vi "YFM11.vi"() -> ()   [LabVIEW 2017]
uses:
  <vilib>/Analysis/6fits.llb/Curve Fitting Criteria.ctl
  <vilib>/DAQmx/write.llb/DAQmx Write (Analog DBL 1Chan 1Samp).vi
  <vilib>/DAQmx/read.llb/DAQmx Read (Analog Wfm 1Chan NSamp).vi
  <vilib>/DAQmx/create/channels.llb/DAQmx Create Channel (AO-Voltage-Basic).vi
  <vilib>/DAQmx/create/channels.llb/DAQmx Create Channel (AI-Voltage-Basic).vi
  <vilib>/DAQmx/configure/timing.llb/DAQmx Timing (Sample Clock).vi
  <vilib>/DAQmx/miscellaneous.llb/DAQmx Fill In Error Info.vi
  <vilib>/Analysis/6fits.llb/1D B-Spline Fit.vi
  <vilib>/Analysis/NI_AALPro.lvlib
panel:
  in  "averaging points":i32=100
  in  "sensitivity^-1":dbl=1000.0
  out "(log)Id(Vg)":cluster{dbl[], "Best BSpline Fit Y":dbl[]}(graph)
  out "intercept":dbl=nan
  out "theta avg.":dbl
  in  "stop":dbl=1.39
  in  "start":dbl=1.39
  out "theta":dbl[](array[numeric])
  in  "theta0":dbl
  out "Rct":dbl=nan
  out "YFM":dbl[](array[numeric])
  out "Vg":dbl[](array[numeric])
  in  "stop":dbl=1.4
  in  "start":dbl=1.1
  out "(Gm)^1/2":dbl=nan
  out "Vt":dbl=nan
  out "theta":cluster{dbl[], dbl[]}(graph)={[0.8, 0.81, 0.8200000000000001, 0.8300000000000001, 0.8400000000000001], [nan, nan, nan, nan, nan]}
  out "YFM":cluster{dbl[], "Best Linear Fit":dbl[]}(graph)
  out "gm":cluster{dbl[], dbl[]}(graph)={[0.8, 0.81, 0.8200000000000001, 0.8300000000000001, 0.8400000000000001], [-1.462188767798153e-07, 1.7166614532470683e-06, 3.266596794128415e-06, 2.5996923446655253e-06, -6.398235458925546e-08]}
  out "Id Array":dbl[](array[numeric])=[-1.173257827758789e-07, -1.1843729019165039e-07, -8.29925537109375e-08, -5.3105354309082036e-08, -3.099870681762695e-08]
  out "Vg Array":dbl[](array[numeric])=[0.8, 0.81, 0.8200000000000001, 0.8300000000000001, 0.8400000000000001]
  in  "Vd":dbl=0.1
  in  "Vd channels":tag="Dev3/ao1"
  in  "Id channels":tag="Dev9/ai0"
  out "# of step":dbl=60.999999999999986
  in  "Step":dbl=0.01
  in  "Stop (V)":dbl=1.4
  in  "Start (V)":dbl=0.8
  in  "Vg channels":tag="Dev3/ao0"
  # "<theta range>"
  # "<linear region>"
  # "Vg"
  # "Fitting"
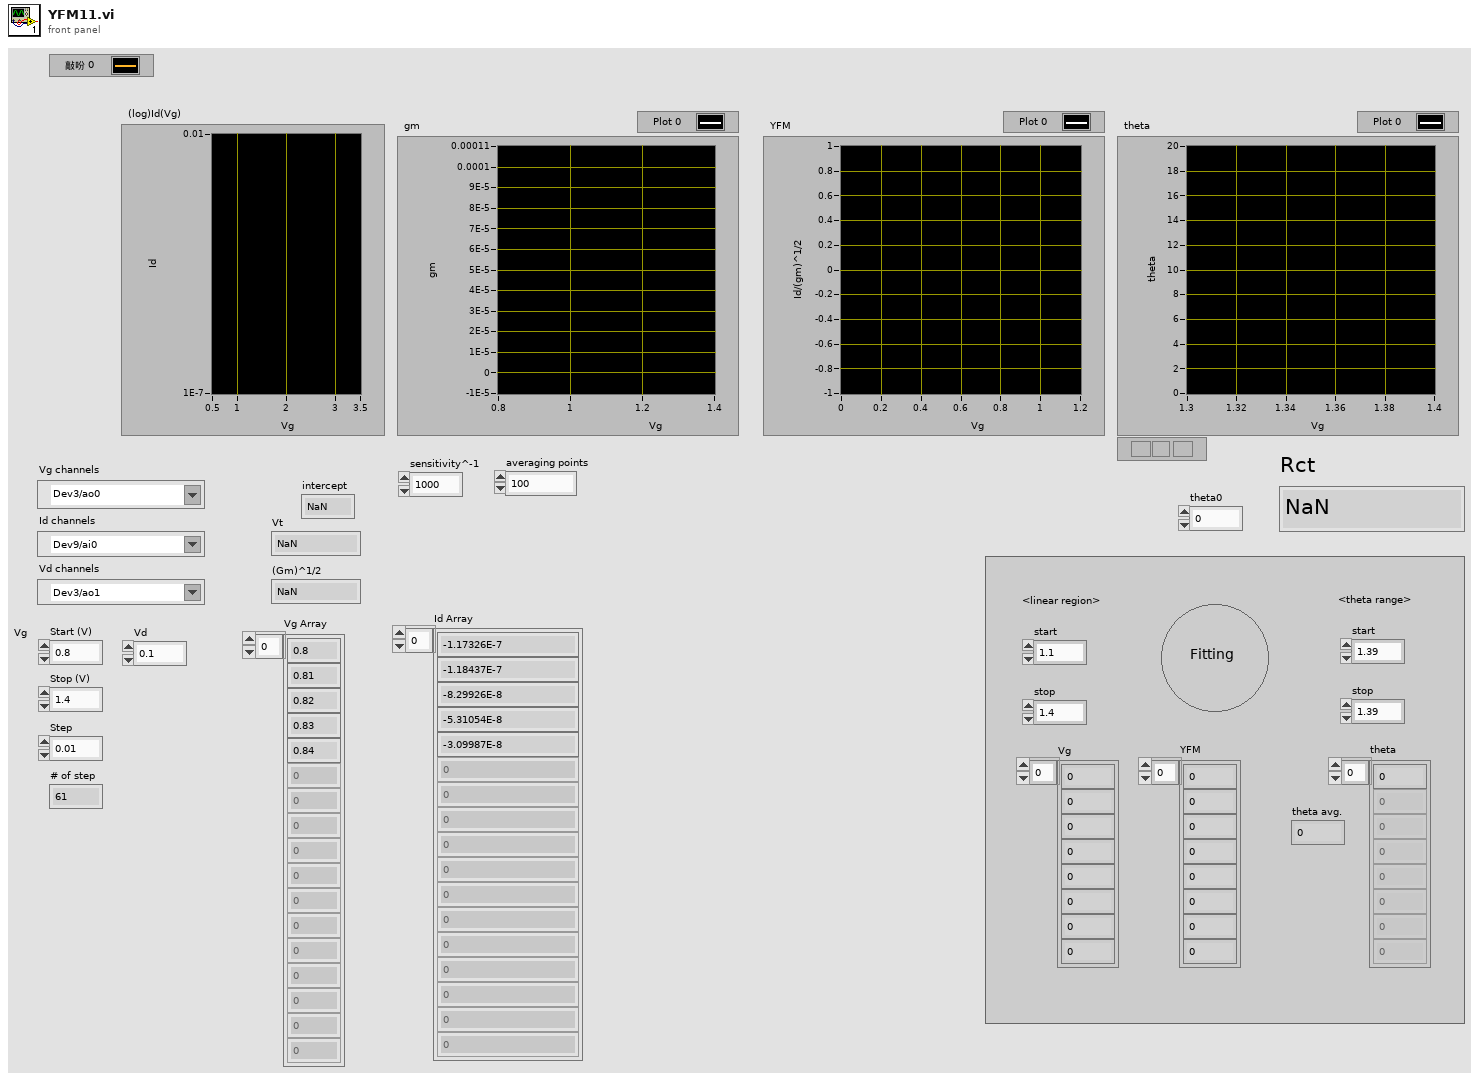
[diagram p1: front panel]
types:
  T1 = typedef "NI_AALPro.lvlib/Curve Fitting Criteria.ctl" = u16
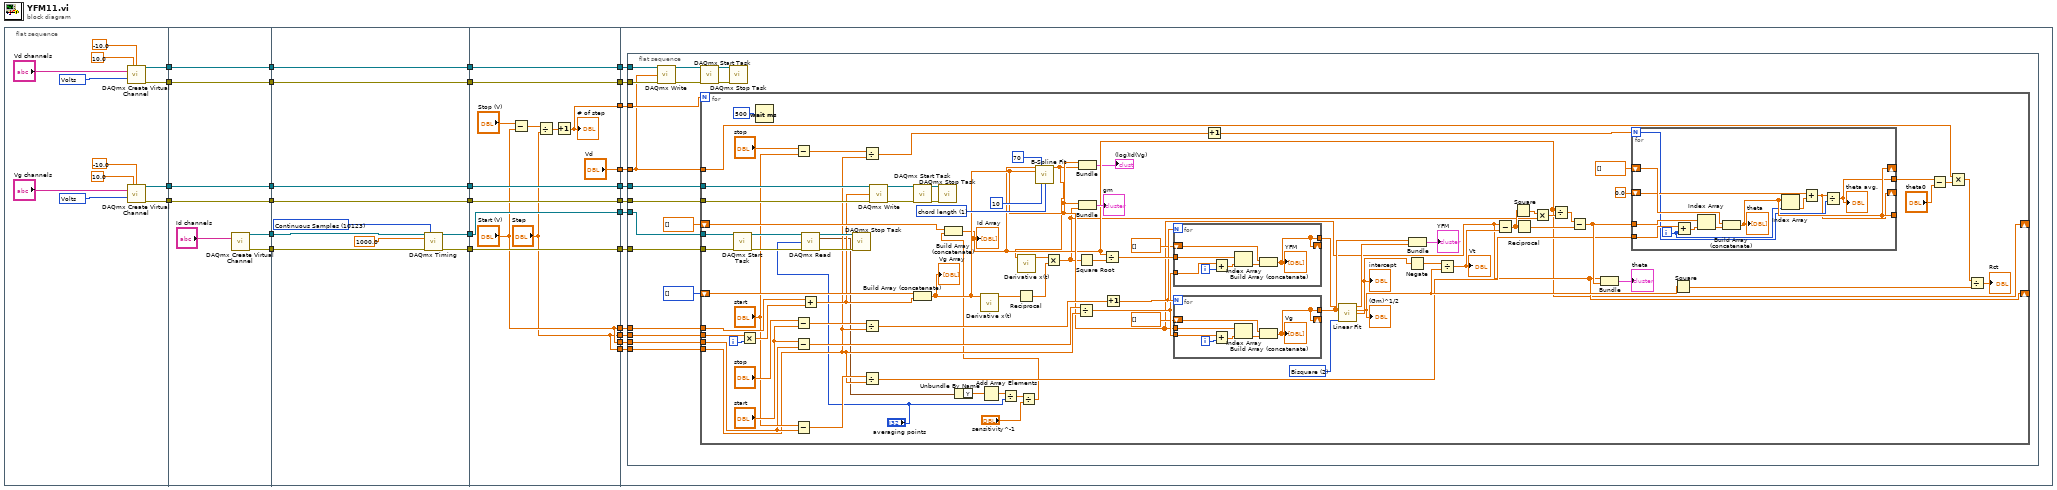
[diagram p0: block diagram]
diagram:
  n1 = flat-sequence {
    tunnel: [w36] -> w18
    tunnel: [w35] -> w16
    tunnel: [w30] -> w8
    tunnel: [w29] -> w4
    tunnel: w18 -> [w47]
    tunnel: [w47] -> w17
    tunnel: w16 -> [w46]
    tunnel: [w46] -> w15
    tunnel: [w44] -> w14
    tunnel: [w43] -> w13
    tunnel: [w42] -> w9
    tunnel: w8 -> [w42]
    tunnel: [w41] -> w5
    tunnel: w4 -> [w41]
    tunnel: w17 -> [w57]
    tunnel: w15 -> [w56]
    tunnel: w14 -> [w55]
    tunnel: w13 -> [w52]
    tunnel: [w57] -> w28
    tunnel: [w56] -> w27
    tunnel: [w51] -> w26
    tunnel: [w50] -> w25
    tunnel: [w49] -> w10
    tunnel: w9 -> [w49]
    tunnel: [w48] -> w6
    tunnel: w5 -> [w48]
    tunnel: w28 -> [w70]
    tunnel: w27 -> [w69]
    tunnel: w26 -> [w68]
    tunnel: w25 -> [w67]
    tunnel: [w70] -> w24
    tunnel: [w69] -> w23
    tunnel: [w68] -> w22
    tunnel: [w67] -> w21
    tunnel: ["Step"] -> w20
    tunnel: ["Start (V)"] -> w19
    tunnel: ["Vd"] -> w12
    tunnel: [w63] -> w11
    tunnel: w10 -> [w63]
    tunnel: [w62] -> w7
    tunnel: w6 -> [w62]
    tunnel: [w60] -> w3
    tunnel: ["Start (V)"] -> w2
    tunnel: ["Step"] -> w1
    tunnel: w24 -> [w80]
    tunnel: w23 -> [w79]
    tunnel: w22 -> [w78]
    tunnel: w21 -> [w77]
    tunnel: w20 -> [w82]
    tunnel: w19 -> [w81]
    tunnel: w12 -> [w76]
    tunnel: w11 -> [w75]
    tunnel: w7 -> [w74]
    tunnel: w3 -> [w73]
    tunnel: w2 -> [w72]
    tunnel: w1 -> [w71]
    frame #0 {
      w32 = 10348 items=["Volts"=10348, "From Custom Scale"=10065] ("units")
      w37 = 10348 items=["Volts"=10348, "From Custom Scale"=10065] ("units")
      n2 = call-poly <vilib>:"DAQmx Create Virtual Channel.vi"("maximum value"=10.0, "minimum value"=-10.0, "physical channels"="Vd channels", "units"=w32) -> ("task out"=w30:refnum<k21>, "error out"=w29:errorcluster)  [unwired: 10 in]
      n3 = call-poly <vilib>:"DAQmx Create Virtual Channel.vi"("maximum value"=10.0, "minimum value"=-10.0, "physical channels"="Vg channels", "units"=w37) -> ("task out"=w36:refnum<k21>, "error out"=w35:errorcluster)  [unwired: 10 in]
    }
    frame #1 {
      n4 = call-poly <vilib>:"DAQmx Create Virtual Channel.vi"("physical channels"="Id channels") -> ("task out"=w44:refnum<k21>, "error out"=w43:errorcluster)  [unwired: 13 in]
    }
    frame #2 {
      w54 = 10123 items=["Finite Samples"=10178, "Continuous Samples"=10123, "Hardware Timed Single Point"=12522] ("sample mode")
      n5 = call-poly <vilib>:"DAQmx Timing.vi"("task/channels in"=w55, "sample mode"=w54, "rate"=1000.0, "error in"=w52) -> ("task out"=w51:refnum<k21>, "error out"=w50:errorcluster)  [unwired: 10 in]
    }
    frame #3 {
      n6 = Subtract(x="Stop (V)", y="Start (V)") -> (x-y=w66:dbl)
      n7 = Divide(x=w66, y="Step") -> (x/y=w61:dbl)
      n8 = Increment(x=w61) -> (x+1=w60:dbl)
      "# of step" <- w60
    }
    frame #4 {
      n9 = flat-sequence {
        tunnel: w82 -> [w93]
        tunnel: w81 -> [w94]
        tunnel: w76 -> [w83]
        tunnel: w75 -> [w98]
        tunnel: w74 -> [w97]
        tunnel: w73 -> [w92]
        tunnel: w78 -> [w91]
        tunnel: w77 -> [w90]
        tunnel: w80 -> [w89]
        tunnel: w79 -> [w88]
        tunnel: w72 -> [w85]
        tunnel: w71 -> [w84]
        frame #0 {
          n10 = call-poly <vilib>:"DAQmx Write.vi"("task/channels in"=w98, "data"=w83, "error in"=w97) -> ("task out"=w100:refnum<k21>, "error out"=w96:errorcluster)  [unwired: 10 in, 1 out]
          n11 = call <vilib>:"DAQmx Start Task.vi"("task/channels in"=w100, "error in"=w96) -> ("task out"=w99:refnum<k21>, "error out"=w95:errorcluster)  [unwired: 12 in]
          n12 = for {
            N: w92 -> [_]
            tunnel: w94 -> [w183]
            tunnel: w93 -> [w182]
            tunnel: w91 -> [w180]
            tunnel: w90 -> [w181]
            tunnel: w89 -> [w175]
            tunnel: w88 -> [w174]
            shift-right: [w112] -> _
            shift-left: i32[] [] -> [w168]
            shift-right: [w111] -> _
            shift-left: dbl[] [] -> [w167]
            tunnel: w85 -> [w120]
            tunnel: w84 -> [w118]
            tunnel: w83 -> [w138]
            i -> [w169]
            w113 = u16 1 items=["equally spaced", "chord length", "centripetal"] ("parameter selection")
            w144 = T1 2 items=["Least Square", "Least Absolute Residual", "Bisquare"] ("method")
            n13 = call <vilib>:"DAQmx Start Task.vi"("task/channels in"=w180, "error in"=w181) -> ("task out"=w179:refnum<k21>, "error out"=w178:errorcluster)  [unwired: 12 in]
            n14 = Multiply(x=w182, y=w169) -> (x*y=w184:dbl)
            n15 = Wait (ms)(milliseconds to wait=u32 500) -> ()  [unwired: 1 out]
            n16 = Subtract(x="stop", y="start") -> (x-y=w134:dbl)
            n17 = Subtract(x="stop", y="start") -> (x-y=w155:dbl)
            n18 = Subtract(x="start", y=w120) -> (x-y=w152:dbl)
            n19 = Subtract(x="start", y=w120) -> (x-y=w119:dbl)
            n20 = call-poly <vilib>:"DAQmx Read.vi"("task/channels in"=w179, "number of samples per channel"="averaging points", "error in"=w178) -> ("task out"=w176:refnum<k21>, "data"=w103:waveform(dbl), "error out"=w177:errorcluster)  [unwired: 10 in]
            n21 = Add(x=w183, y=w184) -> (x+y=w161:dbl)
            n22 = call <vilib>:"DAQmx Stop Task.vi"("task/channels in"=w176, "error in"=w177) -> ()  [unwired: 12 in, 2 out]
            n23 = Divide(x=w134, y=w118) -> (x/y=w133:dbl)
            n24 = Divide(x=w155, y=w118) -> (x/y=w154:dbl)
            n25 = Divide(x=w119, y=w118) -> (x/y=w117:dbl)
            n26 = call-poly <vilib>:"DAQmx Write.vi"("task/channels in"=w175, "data"=w161, "error in"=w174) -> ("task out"=w173:refnum<k21>, "error out"=w172:errorcluster)  [unwired: 10 in, 1 out]
            n27 = call <vilib>:"DAQmx Start Task.vi"("task/channels in"=w173, "error in"=w172) -> ("task out"=w171:refnum<k21>, "error out"=w170:errorcluster)  [unwired: 12 in]
            n28 = Build Array (concatenate)(w168, w161) -> (w112:dbl[])
            "Vg Array" <- w112
            n29 = call <vilib>:"DAQmx Stop Task.vi"("task/channels in"=w171, "error in"=w170) -> ()  [unwired: 12 in, 2 out]
            n30 = Unbundle By Name(w103) -> ("Y"=w104:dbl[])
            n31 = call <vilib>:"Derivative x(t).vi"("X"=w112) -> ("dX/dt"=w164:dbl[])  [unwired: 9 in, 1 out]
            n32 = Add Array Elements(numeric array=w104) -> (sum=w105:dbl)
            n33 = Divide(x=w105, y="averaging points") -> (x/y=w106:dbl)
            n34 = Reciprocal(x=w164) -> (1/x=w163:dbl[])
            n35 = Divide(x=w106, y="sensitivity^-1") -> (x/y=w101:dbl)
            n36 = Build Array (concatenate)(w167, w101) -> (w111:dbl[])
            "Id Array" <- w111
            n37 = call-poly <vilib>:"B-Spline Fit.vi"("Y"=w111, "# of control points"=70, "X"=w112, "degree"=10, "parameter selection"=w113) -> ("Best BSpline Fit Y"=w110:dbl[])  [unwired: 7 in, 3 out]
            n38 = call <vilib>:"Derivative x(t).vi"("X"=w110) -> ("dX/dt"=w165:dbl[])  [unwired: 9 in, 1 out]
            n39 = Multiply(x=w165, y=w163) -> (x*y=w109:dbl[])
            n40 = Divide(x=w152, y=w118) -> (x/y=w145:dbl)
            n41 = Square Root(x=w109) -> (sqrt(x)=w162:dbl[])
            n42 = Bundle(w112, "Best BSpline Fit Y"=w110) -> (→"(log)Id(Vg)":cluster{dbl[], "Best BSpline Fit Y":dbl[]})  [unwired: 1 in]
            n43 = Bundle(w112, w109) -> (→"gm":cluster{dbl[], dbl[]})  [unwired: 1 in]
            n44 = Divide(x=w111, y=w162) -> (x/y=w147:dbl[])
            n45 = Increment(x=w154) -> (x+1=w146:dbl)
            n46 = for {
              N: w146 -> [_]
              shift-right: [w198] -> _
              shift-left: dbl[] [] -> [w200]
              tunnel: w147 -> [w199]
              tunnel: [w198] -> w148
              tunnel: w145 -> [w197]
              i -> [w202]
              n47 = Add(x=w197, y=w202) -> (x+y=w203:dbl)
              n48 = Index Array(array=w199, index=w203) -> (element=w201:dbl)
              n49 = Build Array (concatenate)(w200, w201) -> (w198:dbl[])
              "YFM" <- w198
            }
            n50 = for {
              N: w146 -> [_]
              shift-right: [w205] -> _
              shift-left: dbl[] [] -> [w207]
              tunnel: w112 -> [w206]
              tunnel: [w205] -> w149
              tunnel: w145 -> [w204]
              i -> [w209]
              n51 = Add(x=w204, y=w209) -> (x+y=w210:dbl)
              n52 = Index Array(array=w206, index=w210) -> (element=w208:dbl)
              n53 = Build Array (concatenate)(w207, w208) -> (w205:dbl[])
              "Vg" <- w205
            }
            n54 = Increment(x=w133) -> (x+1=w128:dbl)
            n55 = call <vilib>:"Linear Fit.vi"("Y"=w148, "X"=w149, "method"=w144) -> ("Best Linear Fit"=w151:dbl[], "slope"=w124:dbl, "intercept"=w125:dbl)  [unwired: 8 in, 2 out]
            "(Gm)^1/2" <- w124
            "intercept" <- w125
            n56 = Negate(x=w125) -> (-x=w123:dbl)
            n57 = Bundle(w149, "Best Linear Fit"=w151) -> (→"YFM":cluster{dbl[], "Best Linear Fit":dbl[]})  [unwired: 1 in]
            n58 = Divide(x=w123, y=w124) -> (x/y=w122:dbl)
            "Vt" <- w122
            n59 = Subtract(x=w112, y=w122) -> (x-y=w160:dbl[])
            n60 = Square(x=w160) -> (x^2=w159:dbl[])
            n61 = Reciprocal(x=w160) -> (1/x=w140:dbl[])
            n62 = Multiply(x=w159, y=w109) -> (x*y=w158:dbl[])
            n63 = Divide(x=w111, y=w158) -> (x/y=w141:dbl[])
            n64 = Subtract(x=w141, y=w140) -> (x-y=w132:dbl[])
            n65 = Bundle(w112, w132) -> (→"theta":cluster{dbl[], dbl[]})  [unwired: 1 in]
            n66 = for {
              N: w128 -> [w187]
              shift-right: [w191] -> _
              shift-left: dbl[] [] -> [w194]
              tunnel: w132 -> [w193]
              tunnel: [w191] -> _
              tunnel: w117 -> [w192]
              shift-right: [w186] -> _
              shift-left: 0.0 -> [w189]
              tunnel: [w185] -> w130
              i -> [w190]
              n67 = Add(x=w192, y=w190) -> (x+y=w196:dbl)
              n68 = Index Array(array=w193, index=w196) -> (element=w195:dbl)
              n69 = Build Array (concatenate)(w194, w195) -> (w191:dbl[])
              "theta" <- w191
              n70 = Index Array(array=w191, index=w190) -> (element=w188:dbl)
              n71 = Add(x=w189, y=w188) -> (x+y=w186:dbl)
              n72 = Divide(x=w186, y=w187) -> (x/y=w185:dbl)
              "theta avg." <- w185
            }
            n73 = Square(x=w124) -> (x^2=w126:dbl)
            n74 = Subtract(x=w130, y="theta0") -> (x-y=w137:dbl)
            n75 = Multiply(x=w138, y=w137) -> (x*y=w136:dbl)
            n76 = Divide(x=w136, y=w126) -> (x/y=→"Rct":dbl)
          }
          n77 = call <vilib>:"DAQmx Stop Task.vi"("task/channels in"=w99, "error in"=w95) -> ()  [unwired: 12 in, 2 out]
        }
      }
    }
  }
